vi "PBcard_start.vi"(1 "Bytes/Word":u8=10, 2 "Memory":bool=TRUE, 3 "error in (no error)":errorcluster, 4 "Select Board\nIndicator":i32) -> (7 "error out":errorcluster)   [LabVIEW 2013, in "PulseBlaster.lvlib"]
doc: "This vi sends a software trigger to the PulseBlaster.\n\nIn order to start the PulseBlaster, the following sequence must occur, even if the PulseBlaster is not reprogrammed, but merely retriggered:\n1) Reset the PulseBlaster\n2) Load number of bytes per word\n3) Select Memory device (external or internal)\n4) Clear address counter\n5) Send program finished\n6) Send the \"start\" trigger.\n\nThe inputs should rarely be changed, as they are hardware specific."
uses:
  PulseBlaster.lvlib
  Globals/Total Time.vi
panel:
  # "SOFTWARE TRIGGER"
  # "External"
  # "Internal"
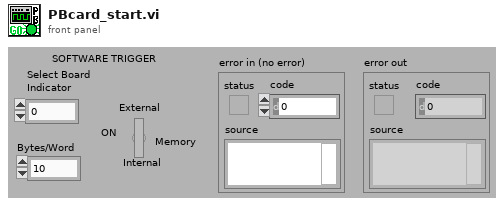
[diagram p1: front panel]
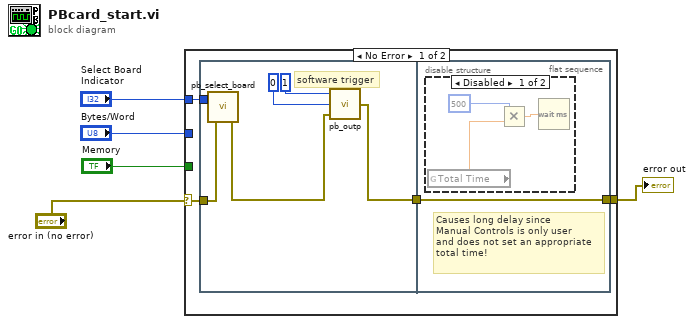
[diagram p0: block diagram]
diagram:
  n1 = case shown="No Error" "error in (no error)" {
    selector: "error in (no error)" -> [w8 w20]
    tunnel: "Bytes/Word" -> [_ _]
    tunnel: "Memory" -> [_ _]
    tunnel: [w7 w20] -> w2
    tunnel: "Select Board\nIndicator" -> [w9 _]
    frame No Error {
      n2 = flat-sequence {
        tunnel: w9 -> [w15]
        tunnel: w8 -> [w14]
        tunnel: [w12] -> w6
        tunnel: [w16] -> w7
        tunnel: w6 -> [w16]
        frame #0 {
          # "software trigger"
          n3 = call "pb_select_board.vi"("error in (no error)"=w14, "Board to Address"=w15) -> ("error out"=w13:errorcluster)
          n4 = call "pb_outp.vi"("error in (no error)"=w13, "8-bit data"=u8 0, "8-bit address offset"=u8 1) -> ("error out"=w12:errorcluster)
        }
        frame #1 {
          # "Causes long delay since\nManual Controls is only user\nand does not set an appropriate\ntotal time!"
          n5 = disable-structure shown="Disabled" {
            frame Disabled {
              n6 = global read "Total Time.vi" "Total Time"() -> (w17:dbl)
              n7 = Multiply(x=500, y=w17) -> (x*y=w19:dbl)
              n8 = Wait (ms)(milliseconds to wait=w19) -> ()  [unwired: 1 out]
            }
            frame Enabled {
            }
          }
        }
      }
    }
    frame Error {
    }
  }
  "error out" <- w2
